vi "Read Latest Record.vi"(7 "TimeStamp Column Name":string, 8 "error in (no error)":errorcluster, 9 "Columns to Read":string[](array[string]), 10 "Table":string, 11 "DatabaseBaseClass in":refnum<class "DatabaseBaseClass.lvclass">) -> (0 "error out":errorcluster, 2 "data":variant[][](array[variant]), 3 "DatabaseBaseClass out":refnum<class "DatabaseBaseClass.lvclass">)   [LabVIEW 2018, in "Database.lvlib" / "DatabaseBaseClass.lvclass"]
uses:
  DatabaseBaseClass.lvclass
  DatabaseBaseClass.lvclass/DatabaseBaseClass.ctl
  <vilib>/addons/database/NI_Database_API.lvlib
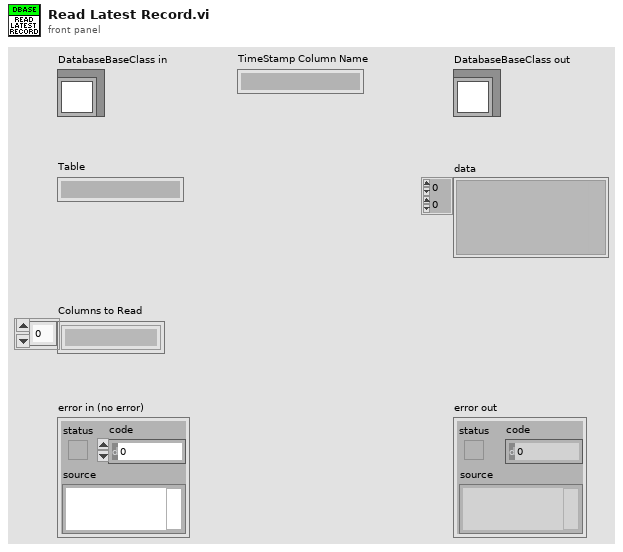
[diagram p1: front panel]
types:
  T1 = typedef "NI_Database_API.lvlib/Conn ObjectReference.ctl" = refnum<k1>
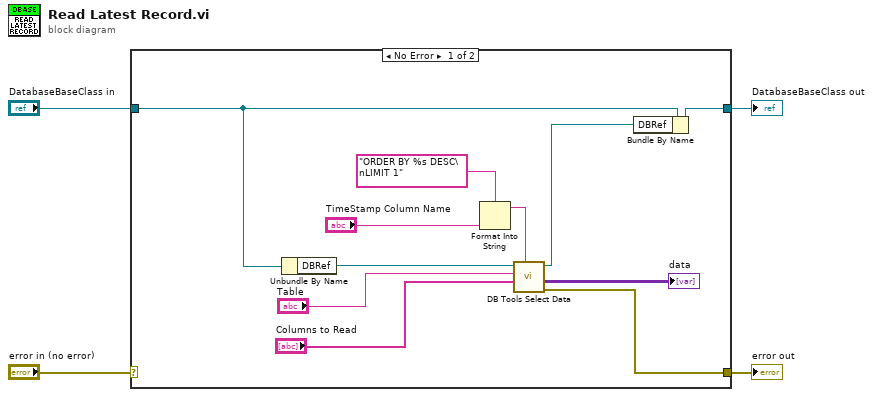
[diagram p0: block diagram]
diagram:
  n1 = case shown="No Error" "error in (no error)" {
    selector: "error in (no error)" -> [_ w17]
    tunnel: [w10 w17] -> w3
    tunnel: [w6 w16] -> w1
    tunnel: "DatabaseBaseClass in" -> [w15 w16]
    frame No Error {
      n2 = Unbundle By Name(w15) -> ("DBRef"=w14:T1)
      n3 = Format Into String(format string="ORDER BY %s DESC\nLIMIT 1", "TimeStamp Column Name") -> (resulting string=w9:string)  [unwired: 2 in, 1 out]
      n4 = call <vilib>:"DB Tools Select Data.vi"("condition"=w9, "columns"="Columns to Read", "table"="Table", "connection reference"=w14) -> ("error out"=w10:errorcluster, "data"=→"data":variant[][], "connection reference out"=w5:T1)  [unwired: 2 in]
      n5 = Bundle By Name(cluster=w15, "DBRef"=w5) -> (w6:refnum<class "DatabaseBaseClass.lvclass">)
    }
    frame Error {
    }
  }
  "error out" <- w3
  "DatabaseBaseClass out" <- w1
